vi "Create Hierarchy Elements.vi"(6 "Hierarchy":string[](array[string]), 9 "Element Map in":map{refnum<class "Config Element.lvclass">, i32}(c390), 10 "Hierarchy Map in":map{string[], i32}(c390), 11 "Elements in":refnum<class "Config Element.lvclass">[](array[class])) -> (0 "error out":errorcluster, 1 "Element Map":map{refnum<class "Config Element.lvclass">, i32}(c390), 2 "Hierarchy Map":map{string[], i32}(c390), 3 "Elements":refnum<class "Config Element.lvclass">[](array[class]), 4 "New Element":refnum<class "Config Element.lvclass">)   [LabVIEW 2023, in "CDM-Config.lvlib" / "Config Manager.lvclass"]
uses:
  Config Manager.lvclass
  Config Element/Config Element.lvclass
  Config Manager.lvclass/Config Manager.ctl
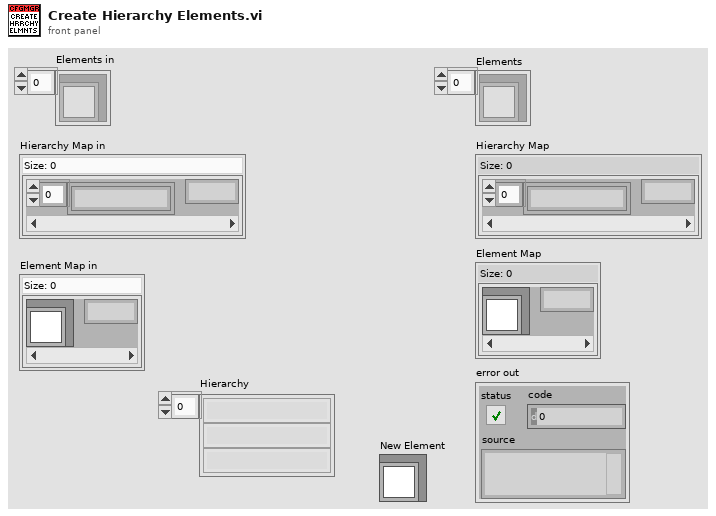
[diagram p1: front panel]
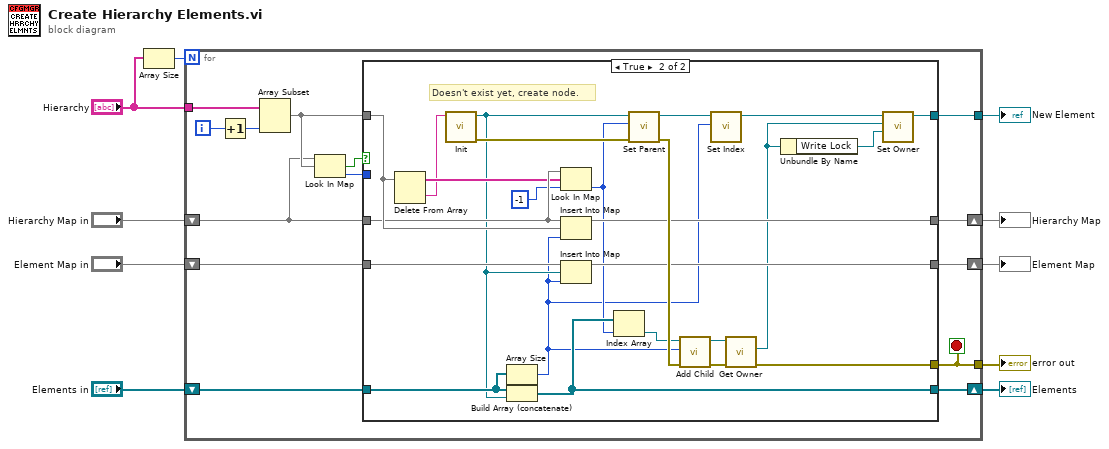
[diagram p0: block diagram]
diagram:
  n1 = Array Size(array="Hierarchy") -> (size(s)=w3:i32)
  n2 = for {
    N: w3 -> [_]
    tunnel: "Hierarchy" -> [w24]
    shift-right: [w14] -> w6
    shift-left: "Hierarchy Map in" -> [w18]
    shift-right: [w15] -> w5
    shift-left: "Element Map in" -> [w20]
    shift-right: [w16] -> w4
    shift-left: "Elements in" -> [w19]
    tunnel: [w12] -> w2
    tunnel: [w11] -> w1
    i -> [w23]
    stop <- w12 stop-if-true
    n3 = Increment(x=w23) -> (x+1=w13:i32)
    n4 = Array Subset(array=w24, length=w13) -> (w21:string[])  [unwired: 1 in]
    n5 = Look In Map(map=w18, key=w21) -> (key not found?=w22:bool, value=w17:i32)  [unwired: 1 in]
    n6 = case shown="True" w22 {
      tunnel: w21 -> [_ w45]
      tunnel: w20 -> [w26 w48]
      tunnel: w19 -> [w25 w49]
      tunnel: w18 -> [w27 w44]
      tunnel: w17 -> [_ _]
      tunnel: [w25 w42] -> w16
      tunnel: [w26 w46] -> w15
      tunnel: [w27 w47] -> w14
      tunnel: [_ w34] -> w12
      tunnel: [_ w33] -> w11
      frame False {
        # "Exists, move on."
      }
      frame True {
        # "Doesn't exist yet, create node."
        n7 = Delete From Array(array=w45) -> (deleted portion=w30:string, array with subset deleted=w43:string[])  [unwired: 2 in]
        n8 = call "Init.vi"("Name"=w30) -> ("error out"=w50:errorcluster, "Config Element out"=w40:refnum<class "Config Element.lvclass">)  [unwired: 9 in]
        n9 = Array Size(array=w49) -> (size(s)=w31:i32)
        n10 = Build Array (concatenate)(w49, w40) -> (w42:refnum<class "Config Element.lvclass">[])
        n11 = Look In Map(map=w44, key=w43, default value=-1) -> (value=w39:i32)  [unwired: 1 out]
        n12 = Insert Into Map(map in=w44, key=w45, value=w31) -> (map out=w47:map{string[], i32})  [unwired: 2 out]
        n13 = Insert Into Map(map in=w48, key=w40, value=w31) -> (map out=w46:map{refnum<class "Config Element.lvclass">, i32})  [unwired: 2 out]
        n14 = Index Array(array=w42, index=w39) -> (element=w41:refnum<class "Config Element.lvclass">)
        n15 = call "Set Parent.vi"("error in (no error)"=w50, "Parent"=w39, "Config Element in"=w40) -> ("error out"=w51:errorcluster, "Config Element out"=w37:refnum<class "Config Element.lvclass">)  [unwired: 7 in]
        n16 = call "Add Child.vi"("error in (no error)"=w51, "Child"=w31, "Config Element in"=w41) -> ("error out"=w35:errorcluster, "Config Element out"=w36:refnum<class "Config Element.lvclass">)  [unwired: 7 in]
        n17 = call "Set Index.vi"("Index"=w31, "Config Element in"=w37) -> ("Config Element out"=w32:refnum<class "Config Element.lvclass">)  [unwired: 8 in, 1 out]
        n18 = call "Get Owner.vi"("error in (no error)"=w35, "Config Element in"=w36) -> ("error out"=w34:errorcluster, "Owner"=w29:refnum<class "Config Manager.lvclass">)  [unwired: 7 in, 1 out]
        n19 = Unbundle By Name(w29) -> ("Write Lock"=w28:refnum<notifier>)
        n20 = call "Set Owner.vi"("Write Lock"=w28, "Owner"=w29, "Config Element in"=w32) -> ("Config Element out"=w33:refnum<class "Config Element.lvclass">)  [unwired: 7 in, 1 out]
      }
    }
  }
  "Hierarchy Map" <- w6
  "Element Map" <- w5
  "Elements" <- w4
  "error out" <- w2
  "New Element" <- w1
